vi "FINAL.vi"() -> ()   [LabVIEW 2018]
uses:
  <vilib>/userdefined/High Color/IMAQdx.ctl
  <vilib>/vision/driver/NI_Vision_Acquisition_Software.lvlib
panel:
  out "Image":T1(plugin-control)
  out "大小 2":i32
  in  "保存照片":bool
  in  "停止":bool
  out "error out":errorcluster
  out "大小":i32
  in  "距离阈值":dbl=900.0 format="%#_13g"
  in  "角度阈值":dbl=30.0 format="%#_13g"
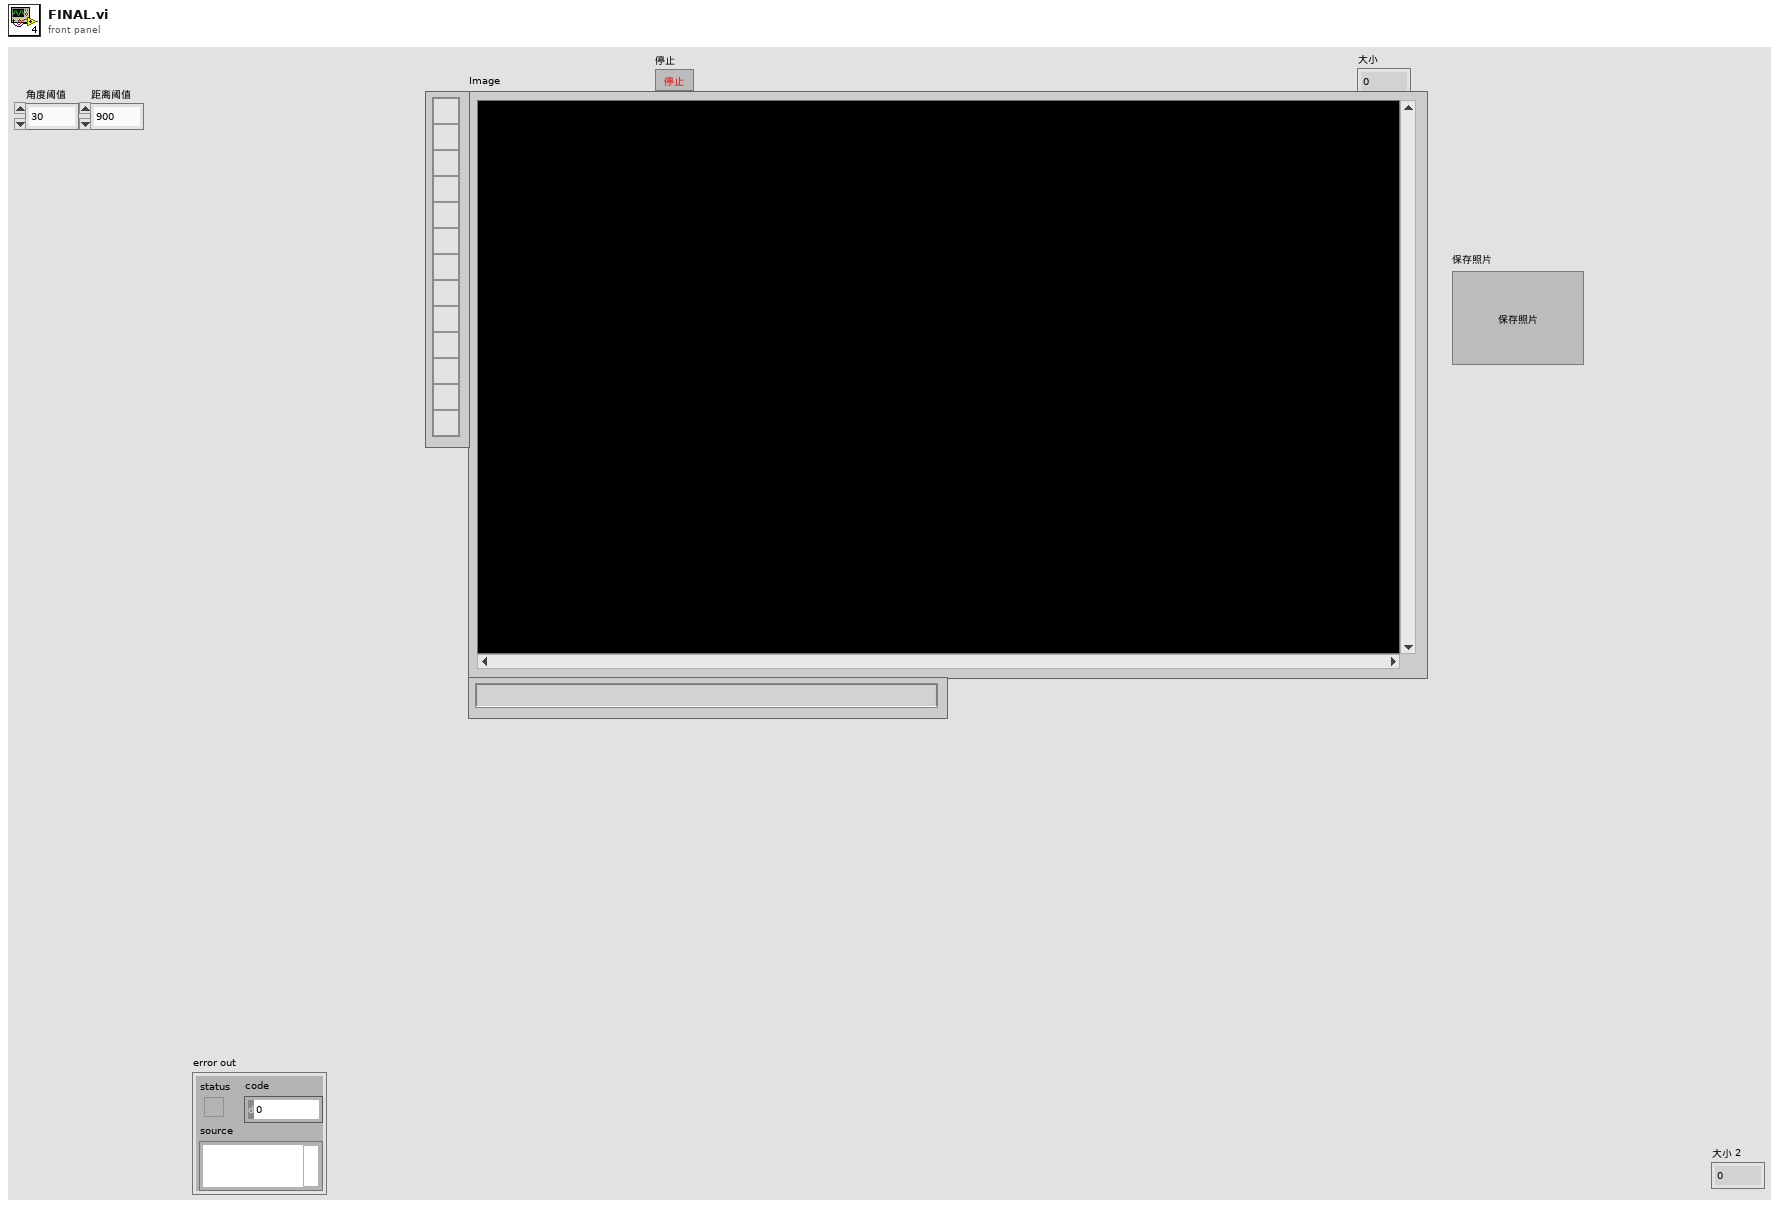
[diagram p1: front panel]
types:
  T1 = typedef "IMAQ Image.ctl" = refnum<image>
  T2 = typedef "IMAQdx.ctl" = refnum<k21>
  T3 = cluster{"Width":u16, "Style":enum32{"Solid", "Dash", "Dot", "DashDot", "DashDotDot"}}
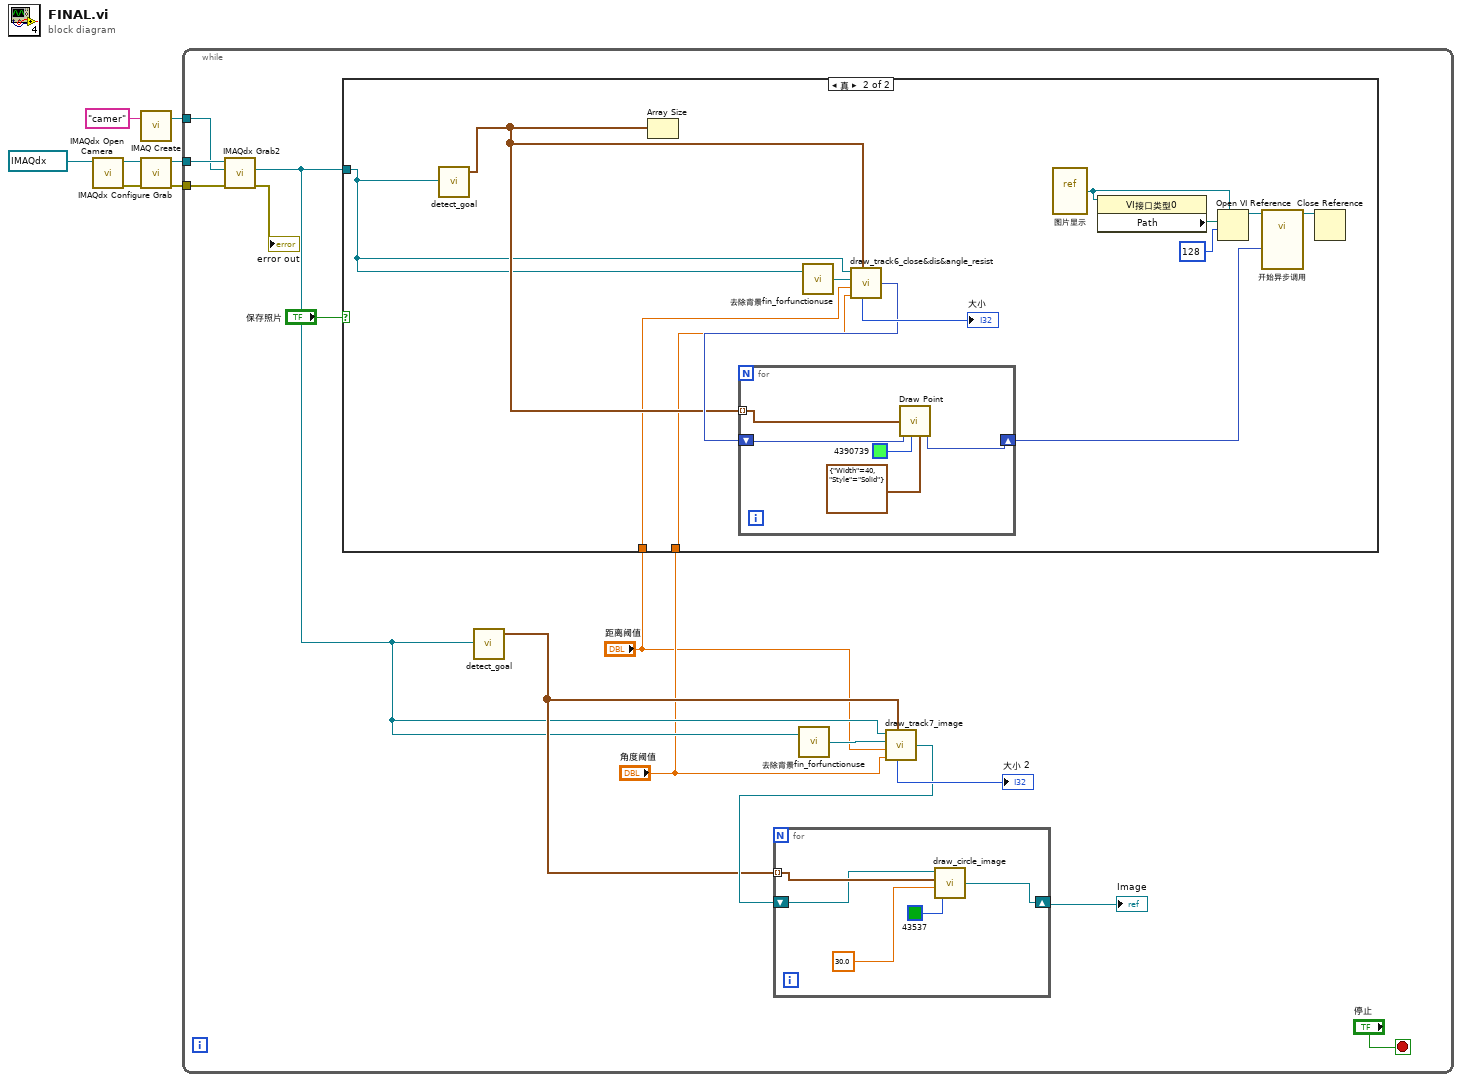
[diagram p0: block diagram]
diagram:
  n1 = call <vilib>:"IMAQdx Open Camera.vi"("Session In"=T2 "cam2") -> ("error out"=w6:errorcluster, "Session Out"=w7:T2)  [unwired: 9 in]
  n2 = call "IMAQ Create"("Image Name"="camer") -> ("New Image"=w4:T1)  [unwired: 4 in, 1 out]
  n3 = call <vilib>:"IMAQdx Configure Grab.vi"("error in"=w6, "Session In"=w7) -> ("error out"=w1:errorcluster, "Session Out"=w5:T2)  [unwired: 8 in]
  n4 = while {
    tunnel: w5 -> [w21]
    tunnel: w4 -> [w20]
    tunnel: w1 -> [w18]
    stop <- "停止" stop-if-true
    n5 = call <vilib>:"IMAQdx Grab2.vi"("error in"=w18, "Image In"=w20, "Session In"=w21) -> ("error out"=→"error out":errorcluster, "Image Out"=w10:T1)  [unwired: 5 in, 2 out]
    n6 = case shown="真" "保存照片" {
      tunnel: w10 -> [_ w29]
      tunnel: "距离阈值" -> [_ w28]
      tunnel: "角度阈值" -> [_ w27]
      frame False {
      }
      frame True {
        n7 = call "detect_goal.vi"("Image Out"=w29) -> ("goal_pos"=w36:cluster{"ave x":dbl, "ave y":dbl}[])  [unwired: 2 out]
        n8 = Array Size(array=w36) -> ()  [unwired: 1 out]
        n9 = call "去除背景fin_forfunctionuse.vi"("Image Src"=w29) -> ("Image Out"=w37:T1)  [unwired: 1 in]
        n10 = call "draw_track6_close&dis&angle_resist.vi"("GOALpos"=w36, "角度阈值"=w27, "距离阈值"=w28, "bin_billard"=w37, "color_billard"=w29) -> ("new picture"=w38:picture, "大小"=→"大小":i32)
        n11 = for {
          tunnel: w36 -> [w41] mode=indexing
          shift-right: [w44] -> w30
          shift-left: w38 -> [w40]
          n12 = call <vilib>:"Draw Point.vi"("picture"=w40, "point(x,y)"=w41, "color(black)"=u32 4390739, "pen"=T3 {"Width"=40, "Style"=enum."Solid"}) -> ("new picture"=w44:picture)  [unwired: 5 in]
        }
        n13 = vi-ref "图片显示.vi"() -> (w35:refnum<vi>)
        n14 = property class="VI接口类型0"(reference=w35) -> ("Path"=w34:path)  [unwired: 1 in, 2 out]
        n15 = Open VI Reference(type specifier VI Refnum (for type only)=w35, vi path=w34, options=128 ("选项")) -> (vi reference=w32:refnum<vi>)  [unwired: 3 in, 1 out]
        n16 = call-by-ref "开始异步调用"(reference=w32, "图片 in"=w30) -> (reference out=w31:refnum<vi>)  [unwired: 2 in, 1 out]
        n17 = Close Reference(reference=w31) -> ()  [unwired: 1 in, 1 out]
      }
    }
    n18 = call "detect_goal.vi"("Image Out"=w10) -> ("goal_pos"=w12:cluster{"ave x":dbl, "ave y":dbl}[])  [unwired: 2 out]
    n19 = call "去除背景fin_forfunctionuse.vi"("Image Src"=w10) -> ("Image Out"=w13:T1)  [unwired: 1 in]
    n20 = call "draw_track7_image.vi"("GOALpos"=w12, "角度阈值"="角度阈值", "距离阈值"="距离阈值", "bin_billard"=w13, "color_billard"=w10) -> ("color_billard 2"=w14:T1, "大小"=→"大小 2":i32)
    n21 = for {
      tunnel: w12 -> [w25] mode=indexing
      shift-right: [w22] -> w11
      shift-left: w14 -> [w23]
      n22 = call "draw_circle_image.vi"("Color"=u32 43537 ("color(black)"), "radius"=30.0, "Position"=w25, "Image"=w23) -> ("Image Out"=w22:T1)
    }
    "Image" <- w11
  }
